vi "VIPM Format build.bat.vi"(8 "error in (no error)":errorcluster, 11 "VIPB File":path) -> (0 "error out":errorcluster, 2 "build.bat Preview":string, 3 "build.bat path":path)   [LabVIEW 2019, in "Build.lvlib"]
uses:
  Build.lvlib
  <vilib>/JKI/VIPM API/command-line/support/VI Package Build Spec Data Cluster_vipm_api.ctl
  <vilib>/JKI/VIPM API/command-line/support/Version Info Cluster_vipm_api.ctl
  <vilib>/JKI/VIPM API/VIPM API_vipm_api.lvlib
panel:
  in  "LV Config":cluster{"LV Version":u32, "Architecture":u32}={"LV Version"=2019, "Architecture"=64} {"Architecture" items=["32"=32, "64"=64]}
  out "Build Spec":T1
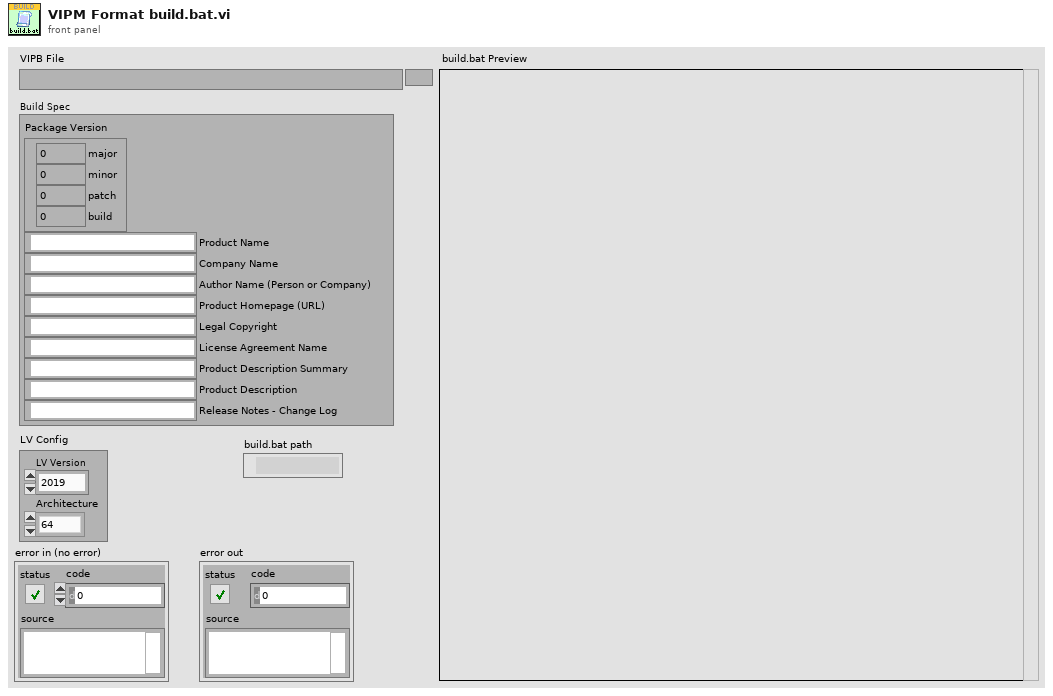
[diagram p1: front panel]
types:
  T1 = typedef "VIPM API_vipm_api.lvlib/VI Package Build Spec Data Cluster_vipm_api.ctl" = cluster{"Package Version":T2, "Product Name":string, "Company Name":string, "Author Name (Person or Company)":string, "Product Homepage (URL)":string, "Legal Copyright":string, "License Agreement Name":string, "Product Description Summary":string, "Product Description":string, "Release Notes - Change Log":string}
  T2 = typedef "VIPM API_vipm_api.lvlib/Version Info Cluster_vipm_api.ctl" = cluster{"major":u32, "minor":u32, "patch":u32, "build":u32}
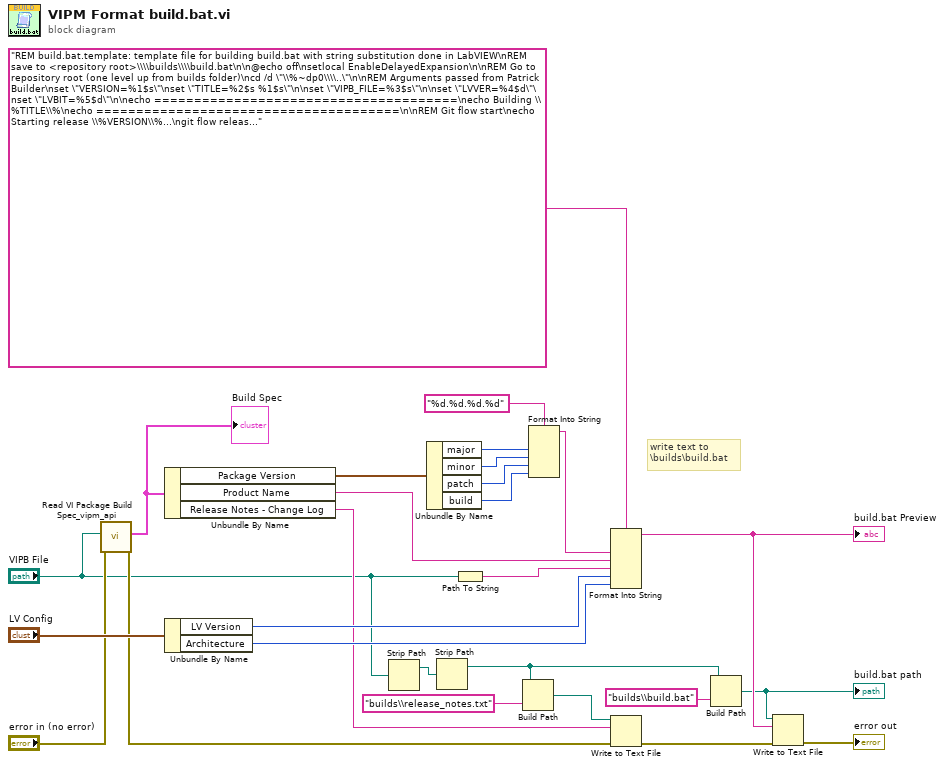
[diagram p0: block diagram]
diagram:
  # "write text to\n\\builds\\build.bat"
  n1 = call <vilib>:"Read VI Package Build Spec_vipm_api.vi"("error in (no error)"="error in (no error)", "Path to VIPB File"="VIPB File") -> ("error out"=w13:errorcluster, "VI Package Build Spec Data"=w2:T1)  [unwired: 8 in]
  "Build Spec" <- w2
  n2 = Unbundle By Name(w2) -> ("Package Version"=w27:T2, "Product Name"=w26:string, "Release Notes - Change Log"=w12:string)
  n3 = Unbundle By Name("LV Config") -> ("LV Version"=w15:u32, "Architecture"=w16:u32)
  n4 = Strip Path(path="VIPB File") -> (stripped path=w8:path)  [unwired: 1 out]
  n5 = Unbundle By Name(w27) -> ("major"=w18:u32, "minor"=w24:u32, "patch"=w23:u32, "build"=w22:u32)
  n6 = Strip Path(path=w8) -> (stripped path=w5:path)  [unwired: 1 out]
  n7 = Path To String(path="VIPB File") -> (string=w20:string)
  n8 = Build Path(base path=w5, name or relative path="builds\\release_notes.txt") -> (appended path=w10:path)
  n9 = Format Into String(format string="%d.%d.%d.%d", w18, w24, w23, w22) -> (resulting string=w21:string)  [unwired: 2 in, 1 out]
  n10 = Format Into String(format string="REM build.bat.template: template file for building build.bat with string substitution done in LabVIEW\nREM save to <repository root>\\\\builds\\\\build.bat\n\n@echo off\nsetlocal EnableDelayedExpansion\n\nREM Go to repository root (one level up from builds folder)\ncd /d \"\\%~dp0\\\\..\"\n\nREM Arguments passed from Patrick Builder\nset \"VERSION=%1$s\"\nset \"TITLE=%2$s %1$s\"\n\nset \"VIPB_FILE=%3$s\"\n\nset \"LVVER=%4$d\"\nset \"LVBIT=%5$d\"\n\necho ======================================\necho Building \\%TITLE\\%\necho ======================================\n\nREM Git flow start\necho Starting release \\%VERSION\\%...\ngit flow release start \\%VERSION\\%\nif \\%ERRORLEVEL\\% neq 0 (\n    echo ERROR: git flow release start failed\n    goto error_handler\n)\n\nREM Archive old releases\necho Archiving previous release...\nif not exist \"builds\\\\old releases\" mkdir \"builds\\\\old releases\"\n\nif exist \"builds\\\\latest\\\\*.*\" (\n    move /Y \"builds\\\\latest\\\\*.*\" \"builds\\\\old releases\\\\\"\n) else (\n    if not exist \"builds\\\\latest\" mkdir \"builds\\\\latest\"\n)\n\nREM Build VIP\necho Building VIP...\ng-cli --lv-ver \\%LVVER\\% --arch \\%LVBIT\\% vipBuild -- \"\\%VIPB_FILE\\%\"\nif \\%ERRORLEVEL\\% neq 0 (\n    echo ERROR: VIP build failed\n    goto error_handler\n)\n\nREM Execute generated launcher script (builds exe/installer/7z)\necho Building executables and installers...\ncall \"builds\\\\7z Install\\\\7zip.bat\"\nif \\%ERRORLEVEL\\% neq 0 (\n    echo ERROR: Executable build failed\n    goto error_handler\n)\n\nREM Git flow finish\necho Committing changes...\ngit commit -m \"Build \\%VERSION\\%\" -a\nif \\%ERRORLEVEL\\% neq 0 (\n    echo ERROR: git commit failed\n    goto error_handler\n)\n\necho Finishing release \\%VERSION\\%...\ngit flow release finish \\%VERSION\\% -m \"Build \\%VERSION\\%\"\nif \\%ERRORLEVEL\\% neq 0 (\n    echo ERROR: git flow release finish failed\n    goto error_handler\n)\n\ngit reset --hard\nif \\%ERRORLEVEL\\% neq 0 (\n    echo ERROR: git reset failed\n    exit /b 1\n)\n\necho Pushing to remote...\ngit push --all\nif \\%ERRORLEVEL\\% neq 0 (\n    echo ERROR: git push --all failed\n    exit /b 1\n)\n\ngit push --tags\nif \\%ERRORLEVEL\\% neq 0 (\n    echo ERROR: git push --tags failed\n    exit /b 1\n)\n\nREM GitHub release\necho Creating GitHub release \\%VERSION\\%...\n\nREM Notes written to builds\\release_notes.txt by Patrick Builder\n\nset ASSETS=\nfor \\%\\%F in (builds\\\\latest\\\\*.vip builds\\\\latest\\\\*.exe) do (\n    set ASSETS=!ASSETS! \"\\%\\%F\"\n)\ngh release create \\%VERSION\\% !ASSETS! -t \"\\%TITLE\\%\" -F builds\\\\release_notes.txt\nif \\%ERRORLEVEL\\% neq 0 (\n    echo ERROR: GitHub release creation failed\n    exit /b 1\n)\n\nREM Clean up temp file\ndel builds\\\\release_notes.txt\n\necho.\necho ======================================\necho Build \\%VERSION\\% completed successfully\necho ======================================\nexit /b 0\n\n:error_handler\necho.\necho ==========================================\necho BUILD FAILED - Cleaning up git state\necho ==========================================\n\nREM Try git flow delete first\ngit flow release delete \\%VERSION\\% 2>nul\n\nREM If that didn't work, manual cleanup\ngit checkout develop 2>nul\ngit branch -D release\\%VERSION\\% 2>nul\n\nexit /b 1", w21, w26, w20, w15, w16) -> (resulting string=w3:string)  [unwired: 2 in, 1 out]
  "build.bat Preview" <- w3
  n11 = Write to Text File(file (use dialog)=w10, text=w12, error in=w13) -> (error out=w7:errorcluster)  [unwired: 1 in, 2 out]
  n12 = Build Path(base path=w5, name or relative path="builds\\build.bat") -> (appended path=w1:path)
  "build.bat path" <- w1
  n13 = Write to Text File(file (use dialog)=w1, text=w3, error in=w7) -> (error out=→"error out":errorcluster)  [unwired: 1 in, 2 out]
